vi "HW_GEN - Build Default Module Configuration.vi"(7 "ModInfo":T1, 8 "error in":errorcluster caption="错误输入", 10 "Chan dflt Para in":T6) -> (0 "error out":errorcluster caption="错误输出", 2 "ModuCfg":T3)   [LabVIEW 2016]
uses:
  Ctrls/HardWare _ Channel Configurations PopUp Type.ctl
  ToolKit/Popup/Private/Ctrls/POP_Data Type.ctl
  Ctrls/HardWare _ Module Configuration.ctl
  Gantner/HW_Module Info.ctl
  Ctrls/HardWare Basic Info _ Channel.ctl
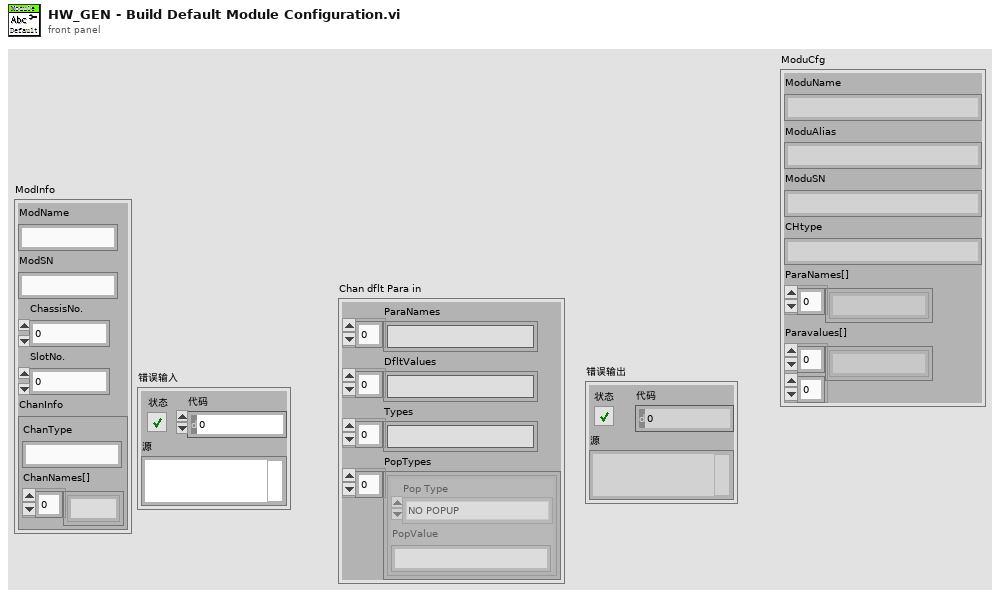
[diagram p1: front panel]
types:
  T1 = typedef "HW_Module Info.ctl" = cluster{"ModName":string, "ModSN":string, "ChassisNo.":u32, "SlotNo.":u32, "ChanInfo":T2}
  T2 = typedef "HardWare Basic Info _ Channel.ctl" = cluster{"ChanType":string, "ChanNames[]":string[]}
  T3 = typedef "HardWare _ Module Configuration.ctl" = cluster{"ModuName":string, "ModuAlias":string, "ModuSN":string, "CHtype":string, "ParaNames[]":string[], "Paravalues[]":string[][]}
  T4 = typedef "HardWare _ Channel Configurations PopUp Type.ctl" = cluster{"Pop Type":T5, "PopValue":string}
  T5 = typedef "POP_Data Type.ctl" = enum16{"NO POPUP", "Unkown", "String", "Integer", "Float", "Color", "Boolean", "Ring", "Captioned String", "Captioned Integer", "Button Color", "2 Int Cluster", "4 Int Cluster", "6-Dbl Cluster", "Path", "Combox", "Time", "ShotCut String"}
  T6 = cluster{"ParaNames":string[], "DfltValues":string[], "Types":string[], "PopTypes":T4[]}
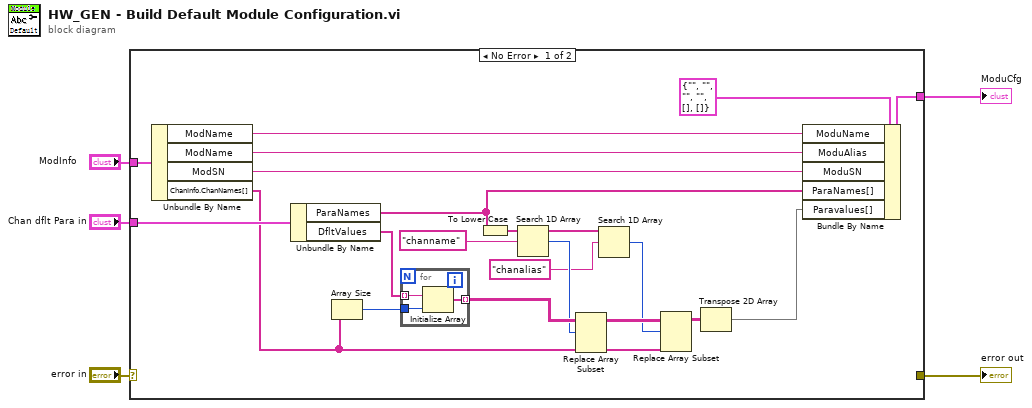
[diagram p0: block diagram]
diagram:
  n1 = case shown="No Error" "error in" {
    selector: "error in" -> [_ w29]
    tunnel: [_ w29] -> w4
    tunnel: "Chan dflt Para in" -> [w25 _]
    tunnel: "ModInfo" -> [w22 _]
    tunnel: [w21 _] -> w1
    frame No Error {
      n2 = Unbundle By Name(w22) -> ("ModName"=w8:string, "ModName"=w9:string, "ModSN"=w10:string, "ChanInfo.ChanNames[]"=w12:string[])
      n3 = Unbundle By Name(w25) -> ("ParaNames"=w7:string[], "DfltValues"=w24:string[])
      n4 = Array Size(array=w12) -> (size(s)=w23:i32)
      n5 = for {
        tunnel: w24 -> [w28] mode=indexing
        tunnel: w23 -> [w27]
        tunnel: [w26] -> w19 mode=indexing
        n6 = Initialize Array(w28, w27) -> (w26:string[])
      }
      n7 = To Lower Case(string=w7) -> (all lower case string=w16:string[])
      n8 = Search 1D Array(1D array=w16, element="channame") -> (index of element=w18:i32)  [unwired: 1 in]
      n9 = Replace Array Subset(array=w19, new element=w12, index (row)=w18) -> (w17:string[][])  [unwired: 1 in]
      n10 = Search 1D Array(1D array=w16, element="chanalias") -> (index of element=w14:i32)  [unwired: 1 in]
      n11 = Replace Array Subset(array=w17, new element=w12, index (row)=w14) -> (w13:string[][])  [unwired: 1 in]
      n12 = Transpose 2D Array(2D array=w13) -> (transposed array=w6:string[][])
      n13 = Bundle By Name(cluster=T3 {"ModuName"="", "ModuAlias"="", "ModuSN"="", "CHtype"="", "ParaNames[]"=[], "Paravalues[]"=[]} ("ModuCfg"), "ModuName"=w8, "ModuAlias"=w9, "ModuSN"=w10, "ParaNames[]"=w7, "Paravalues[]"=w6) -> (w21:T3)
    }
    frame Error {
    }
  }
  "error out" <- w4
  "ModuCfg" <- w1
